vi "13.1 Log Warning (SubVI).vi"(8 "Error In":errorcluster, 10 "Weather Data In":T1, 11 "refnum in":refnum<file>) -> (0 "Error Out":errorcluster, 3 "refnum out":refnum<file>)   [LabVIEW 2019]
uses:
  13.1 Weather Data.ctl
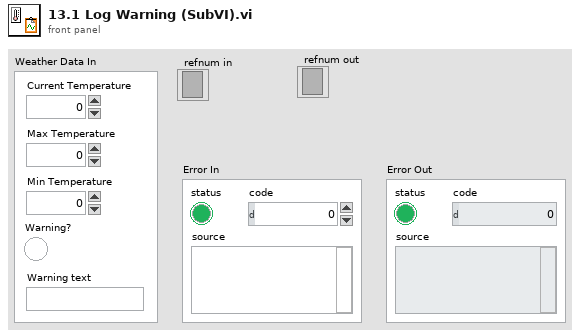
[diagram p1: front panel]
types:
  T1 = typedef "13.1 Weather Data.ctl" = cluster{"Current Temperature":dbl, "Max Temperature":dbl, "Min Temperature":dbl, "Warning?":bool, "Warning text":string}
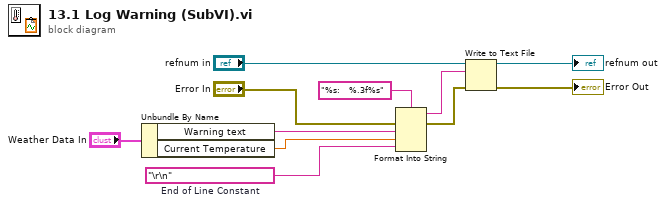
[diagram p0: block diagram]
diagram:
  w7 = "\r\n"  # End of Line Constant
  n1 = Unbundle By Name("Weather Data In") -> ("Warning text"=w2:string, "Current Temperature"=w1:dbl)
  n2 = Format Into String "Format Into String"(format string="%s:   %.3f%s", error in="Error In", w2, w1, w7) -> (resulting string=w11:string, error out=w10:errorcluster)  [unwired: 1 in]
  n3 = Write to Text File(file (use dialog)="refnum in", text=w11, error in=w10) -> (refnum out=→"refnum out":refnum<file>, error out=→"Error Out":errorcluster)  [unwired: 1 in, 1 out]
